vi "64x48_Frame2.vi"   [LabVIEW 2014]
uses:
  QwaveSys_Interface/QwaveSys_Interface.lvlib
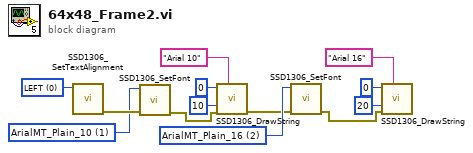
[diagram p0: block diagram]
diagram:
  w5 = u16 2 items=["Crushed_Plain_36", "ArialMT_Plain_10", "ArialMT_Plain_16", "ArialMT_Plain_24"] ("Font")
  w6 = u16 1 items=["Crushed_Plain_36", "ArialMT_Plain_10", "ArialMT_Plain_16", "ArialMT_Plain_24"] ("Font")
  w7 = u16 0 items=["LEFT", "CENTER", "RIGHT"] ("alignment")
  n1 = call "SSD1306_SetTextAlignment.vi"("alignment"=w7) -> ("error out"=w8:errorcluster)  [unwired: 10 in]
  n2 = call "SSD1306_SetFont.vi"("error in (no error)"=w8, "Font"=w6) -> ("error out"=w4:errorcluster)  [unwired: 9 in]
  n3 = call "SSD1306_DrawString.vi"("String"="Arial 10", "error in (no error)"=w4, "y"=u8 10, "x"=u8 0) -> ("error out"=w3:errorcluster)  [unwired: 7 in]
  n4 = call "SSD1306_SetFont.vi"("error in (no error)"=w3, "Font"=w5) -> ("error out"=w2:errorcluster)  [unwired: 9 in]
  n5 = call "SSD1306_DrawString.vi"("String"="Arial 16", "error in (no error)"=w2, "y"=u8 20, "x"=u8 0) -> ()  [unwired: 7 in, 1 out]
